vi "HMI-Reactor.vi"() -> ()   [LabVIEW 2018]
uses:
  <vilib>/Modbus/master/Create Master Instance (TCP).vi
  <vilib>/Modbus/master/Modbus Master.lvclass
panel:
  in  "type":u16[](array[numeric])
  in  "cast type 2":dbl[](array[numeric])
  out "F":dbl
  in  "cast type":dbl[](array[numeric])
  out "CA":dbl=456.3558684423593 format="%#_3g"
  out "CA0":dbl=2000.0 format="%#_3g"
  out "10SDV502":bool=TRUE
  out "?":dbl format="%#_3g"
  in  "10HIC300":dbl=50.0
  out "TJ":dbl=365.3749789937039 format="%#_3g"
  out "T":dbl=333.97788169438996 format="%#_3g"
  out "Reactor Temp":T1={"% Opening"=0.0, "SP"=0.0, "Reactor Temp"=333.97788169438996, "Temp"=333.97788169438996} {"Temp" format="%#_4g"; "Reactor Temp" scale=0.0..700.0; "SP" scale=0.0..700.0; "% Opening" scale=0.0..100.0}
  in  "10TIC100 Faceplate":T2={"PID Parameters"={"KP"=1.0, "KI"=0.01, "KD"=0.0}, "M"=FALSE, "SP_VAL"=0.0, "% Open"=50.0}
  out "?":dbl format="%#_3g"
  out "10SDV501":bool=TRUE
  out "FJ":dbl=15.0 format="%#_3g"
  out "TJ0":dbl=300.0 format="%#_3g"
  out "10SDV500":bool=TRUE
  out "F0":dbl=1.0 format="%#_3g"
  out "T0":dbl=323.0 format="%#_3g"
  out "Reactor Level":T3={"% Opening"=0.0, "SP"=0.0, "Reactor Level"=54.508701366151044, "Level"=54.508701366151044} {"Level" format="%#_4g"; "Reactor Level" scale=0.0..100.0; "SP" scale=0.0..100.0; "% Opening" scale=0.0..100.0}
  out "?":dbl format="%#_3g"
  in  "10LIC200 Faceplate":T2={"PID Parameters"={"KP"=1.0, "KI"=0.01, "KD"=0.0}, "M"=FALSE, "SP_VAL"=0.0, "% Open"=50.0}
  out "10-R-100":dbl(slide)=54.508701366151044 scale=0.0..100.0 scale format="%#_4g"
  in  "stop":bool
  # "this loop is used to regulate the reactor level"
  # "LIC = level controller"
  # "feed flow"
  # "Reactant inlet concentration"
  # "m3/min"
  # "Mole/m3"
  # "10LV200"
  # "%"
  # "K"
  # "%"
  # "this loop is used to regulate the reactor temperature"
  # "K"
  # "TIC=Temperature controller"
  # "coolant flow"
  # "m3/min"
  # "10TV100"
  # "%"
  # "K"
  # "Mole/m3"
  # "%"
  # "K"
  # "coolant inlet temp"
  # "A"
  # "%"
  # "A"
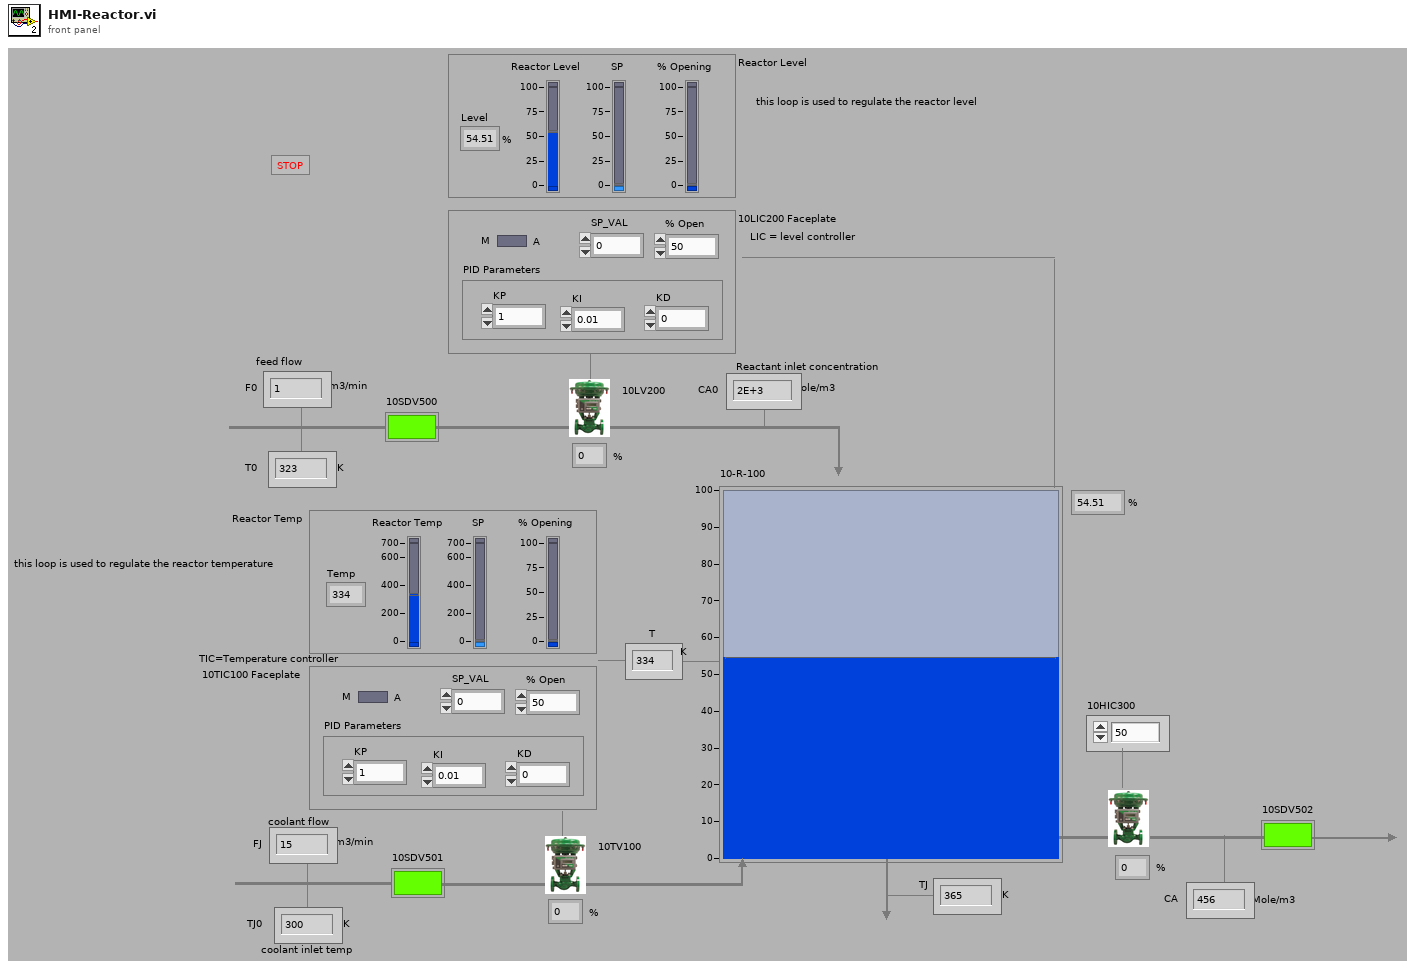
[diagram p1: front panel]
types:
  T1 = cluster{"% Opening":dbl, "SP":dbl, "Reactor Temp":dbl, "Temp":dbl}
  T2 = cluster{"PID Parameters":cluster{"KP":dbl, "KI":dbl, "KD":dbl}, "M":bool, "SP_VAL":dbl, "% Open":dbl}
  T3 = cluster{"% Opening":dbl, "SP":dbl, "Reactor Level":dbl, "Level":dbl}
  T4 = cluster{"% Open":dbl, "SP_VAL":dbl, "Numeric":dbl, "Numeric":dbl}
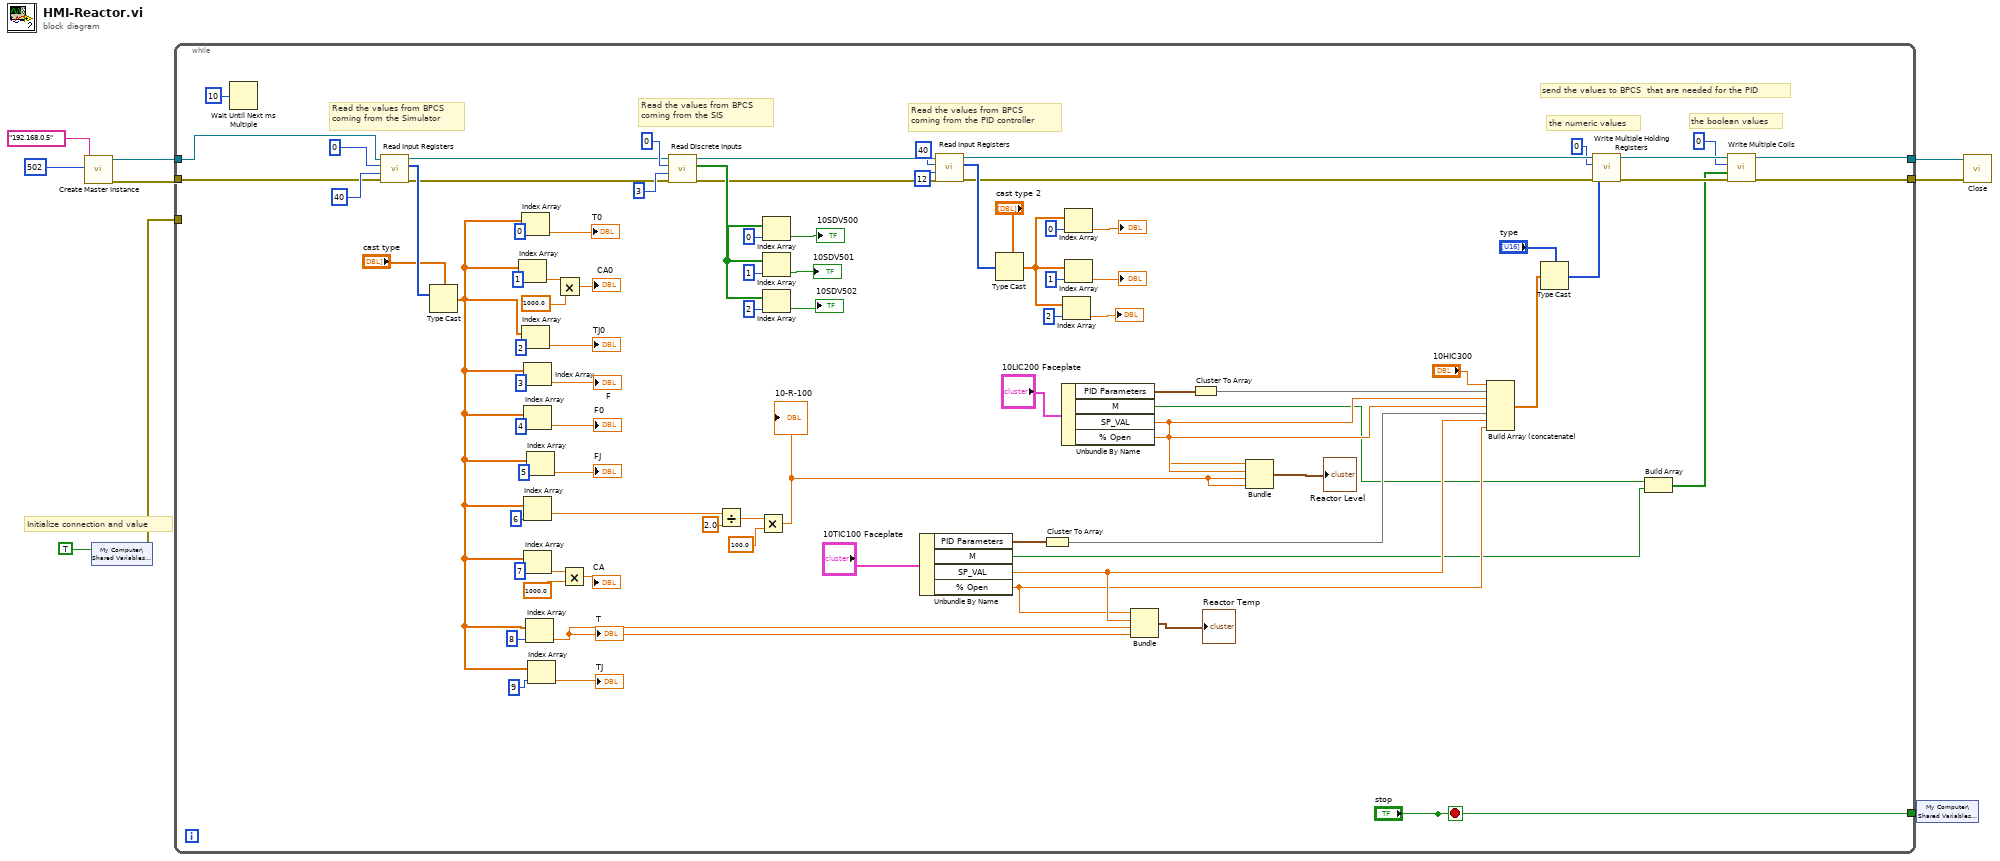
[diagram p0: block diagram]
diagram:
  # "Initialize connection and value"
  n1 = call-poly <vilib>:"Create Master Instance.vi"("port (502)"=u16 502, "address"="192.168.0.5") -> ("error out"=w1:errorcluster, "TCP master instance"=w4:refnum<class "Modbus Master.lvclass">)  [unwired: 8 in]
  n2 = shared-variable "My Computer\\Shared Variables.lvlib\\stop"(TRUE) -> (error out=w8:errorcluster)  [unwired: 1 in]
  n3 = while {
    tunnel: ["stop"] -> w9
    tunnel: w8 -> [_]
    tunnel: w4 -> [w56]
    tunnel: [w11] -> w2
    tunnel: w1 -> [w10]
    tunnel: [w12] -> w3
    stop <- "stop" stop-if-true
    # "the boolean values"
    # "the numeric values"
    # "send the values to BPCS  that are needed for the PID"
    # "Read the values from BPCS \ncoming from the PID controller"
    # "Read the values from BPCS \ncoming from the SIS"
    # "Read the values from BPCS \ncoming from the Simulator"
    n4 = Wait Until Next ms Multiple(millisecond multiple=u32 10) -> ()  [unwired: 1 out]
    n5 = call-dynamic "Read Input Registers.vi"("error in (no error)"=w10, "number of input registers"=u16 40, "starting address"=u16 0, "Modbus master in"=w56) -> ("error out"=w45:errorcluster, "register values"=w84:u16[], "Modbus master out"=w46:refnum<class "Modbus Master.lvclass">)  [unwired: 5 in]
    n6 = Type Cast(type="cast type", x=w84) -> (*(type *) &x=w58:dbl[])
    n7 = Index Array(array=w58, index=1) -> (element=w79:dbl)
    n8 = Index Array(array=w58, index=0) -> (element=→"T0":dbl)
    n9 = Index Array(array=w58, index=2) -> (element=→"TJ0":dbl)
    n10 = Index Array(array=w58, index=3) -> (element=→"F":dbl)
    n11 = Index Array(array=w58, index=6) -> (element=w62:dbl)
    n12 = Index Array(array=w58, index=4) -> (element=→"F0":dbl)
    n13 = Index Array(array=w58, index=7) -> (element=w63:dbl)
    n14 = Index Array(array=w58, index=8) -> (element=w59:dbl)
    "T" <- w59
    n15 = Index Array(array=w58, index=5) -> (element=→"FJ":dbl)
    n16 = Index Array(array=w58, index=9) -> (element=→"TJ":dbl)
    n17 = Multiply(x=w79, y=1000.0) -> (x*y=→"CA0":dbl)
    n18 = Multiply(x=w63, y=1000.0) -> (x*y=→"CA":dbl)
    n19 = call-dynamic "Read Discrete Inputs.vi"("error in (no error)"=w45, "number of discrete inputs"=u16 3, "starting address"=u16 0, "Modbus master in"=w46) -> ("error out"=w43:errorcluster, "discrete input values"=w53:bool[], "Modbus master out"=w44:refnum<class "Modbus Master.lvclass">)  [unwired: 5 in]
    n20 = Divide(x=w62, y=2.0 ("x")) -> (x/y=w94:dbl)
    n21 = Multiply(x=w94, y=100.0) -> (x*y=w83:dbl)
    "10-R-100" <- w83
    n22 = Index Array(array=w53, index=0) -> (element=→"10SDV500":bool)
    n23 = Index Array(array=w53, index=1) -> (element=→"10SDV501":bool)
    n24 = Index Array(array=w53, index=2) -> (element=→"10SDV502":bool)
    n25 = Unbundle By Name("10TIC100 Faceplate") -> ("PID Parameters"=w88:cluster{"KP":dbl, "KI":dbl, "KD":dbl}, "M"=w14:bool, "SP_VAL"=w21:dbl, "% Open"=w20:dbl)
    n26 = call-dynamic "Read Input Registers.vi"("error in (no error)"=w43, "number of input registers"=u16 12, "starting address"=u16 40, "Modbus master in"=w44) -> ("error out"=w30:errorcluster, "register values"=w39:u16[], "Modbus master out"=w31:refnum<class "Modbus Master.lvclass">)  [unwired: 5 in]
    n27 = Type Cast(type="cast type 2", x=w39) -> (*(type *) &x=w38:dbl[])
    n28 = Cluster To Array(cluster=w88) -> (array=w22:dbl[])
    n29 = Unbundle By Name("10LIC200 Faceplate") -> ("PID Parameters"=w91:cluster{"KP":dbl, "KI":dbl, "KD":dbl}, "M"=w15:bool, "SP_VAL"=w24:dbl, "% Open"=w23:dbl)
    n30 = Index Array(array=w38, index=2) -> (element=→"?":dbl)
    n31 = Index Array(array=w38, index=0) -> (element=→"?":dbl)
    n32 = Index Array(array=w38, index=1) -> (element=→"?":dbl)
    n33 = Bundle("% Open"=w20, "SP_VAL"=w21, "Numeric"=w59, "Numeric"=w59) -> (→"Reactor Temp":T4)  [unwired: 1 in]
    n34 = Cluster To Array(cluster=w91) -> (array=w25:dbl[])
    n35 = Bundle("% Open"=w23, "SP_VAL"=w24, w83, w83) -> (→"Reactor Level":cluster{"% Open":dbl, "SP_VAL":dbl, dbl, dbl})  [unwired: 1 in]
    n36 = Build Array (concatenate)("10HIC300", w25, w24, w23, w22, w21, w20) -> (w19:dbl[])
    n37 = Type Cast(type="type", x=w19) -> (*(type *) &x=w28:u16[])
    n38 = call-dynamic "Write Multiple Holding Registers.vi"("error in (no error)"=w30, "holding register values"=w28, "starting address"=u16 0, "Modbus master in"=w31) -> ("error out"=w17:errorcluster, "Modbus master out"=w18:refnum<class "Modbus Master.lvclass">)  [unwired: 6 in]
    n39 = Build Array(w15, w14) -> (w13:bool[])
    n40 = call-dynamic "Write Multiple Coils.vi"("error in (no error)"=w17, "coil values"=w13, "starting address"=u16 0, "Modbus master in"=w18) -> ("error out"=w12:errorcluster, "Modbus master out"=w11:refnum<class "Modbus Master.lvclass">)  [unwired: 6 in]
  }
  n41 = shared-variable "My Computer\\Shared Variables.lvlib\\stop"(w9) -> ()  [unwired: 1 in, 1 out]
  n42 = call-dynamic "Close.vi"("error in (no error)"=w3, "Modbus master in"=w2) -> ()  [unwired: 9 in, 1 out]
